vi "Configure Form Object.vi"(8 "error in (no error)":errorcluster, 10 "Table Name":string, 11 "Panel Form Controller in":refnum<class "Panel Form Controller.lvclass">) -> (0 "error out":errorcluster, 3 "Panel Form Controller out":refnum<class "Panel Form Controller.lvclass">)   [LabVIEW 2020]
uses:
  Database OOP/Table Libraries/Basic Table/Basic Table Class/Basic Table.lvclass
  Database OOP/Table Libraries/Table Configuration Interface/Table Configuration Interface.lvclass
  Panel Form Controller.lvclass
  C:/Program Files (x86)/National Instruments/LabVIEW 2020/vi.lib/MGI/Panel Manager/Panel Actor/Panel Actor/Panel Actor.lvclass
  C:/Program Files (x86)/National Instruments/LabVIEW 2020/vi.lib/MGI/Monitored Actor/Monitored Actor/Monitored Actor/Monitored Actor.lvclass
  C:/Program Files (x86)/National Instruments/LabVIEW 2020/vi.lib/ActorFramework/Actor/Actor.lvclass
  C:/Users/User/Desktop/Raman Program/Database OOP/source/Forms AF/Form Controller/Panel Form Controller.lvclass
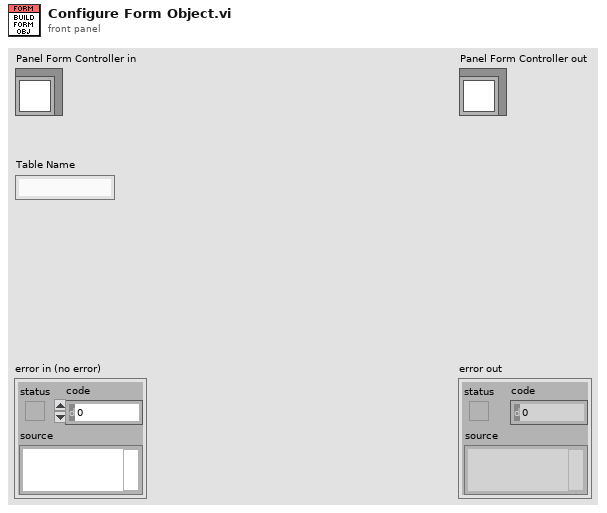
[diagram p1: front panel]
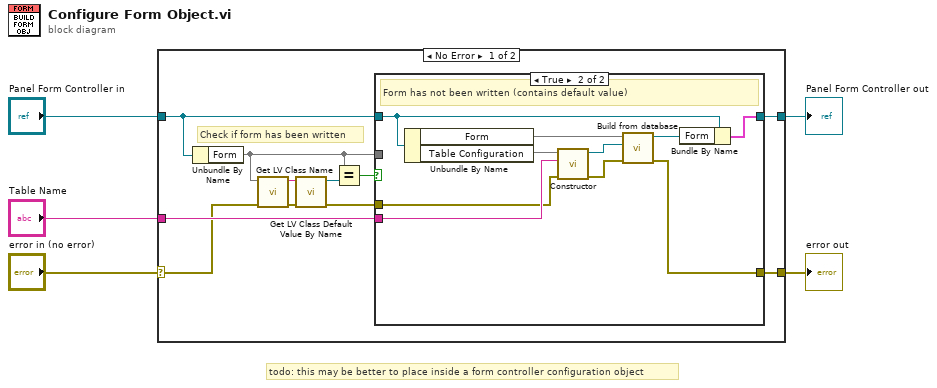
[diagram p0: block diagram]
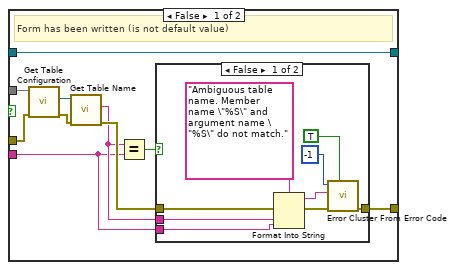
[diagram p2: hidden frame]
diagram:
  # "todo: this may be better to place inside a form controller configuration object"
  n1 = case shown="No Error" "error in (no error)" {
    selector: "error in (no error)" -> [w8 w48]
    tunnel: [w6 w48] -> w4
    tunnel: [w12 w47] -> w2
    tunnel: "Panel Form Controller in" -> [w13 w47]
    tunnel: "Table Name" -> [w10 _]
    frame No Error {
      # "Check if form has been written"
      n2 = Unbundle By Name(w13) -> ("Form"=w9)
      n3 = call <vilib>:"Get LV Class Name.vi"("error in (no error)"=w8, "object"=w9) -> ("error out"=w16:errorcluster, "class name"=w15:string)  [unwired: 8 in]
      n4 = call <vilib>:"Get LV Class Default Value By Name.vi"("error in (no error)"=w16, "class name"=w15) -> ("error out"=w7:errorcluster, "object"=w14:refnum<class>)  [unwired: 8 in]
      n5 = Equal?(x=w9, y=w14) -> (x = y?=w11:bool)
      n6 = case shown="True" w11 {
        tunnel: w13 -> [w24 w46]
        tunnel: [w24 w45] -> w12
        tunnel: w10 -> [w19 w43]
        tunnel: w9 -> [w26 _]
        tunnel: w7 -> [w25 w42]
        tunnel: [w18 w37] -> w6
        frame False {
          # "Form has been written (is not default value)"
          n7 = call "Get Table Configuration.vi"("error in (no error)"=w25, "Basic Table in"=w26) -> ("error out"=w17:errorcluster, "Table Configuration"=w23:refnum<class "Table Configuration Interface.lvclass">)  [unwired: 7 in, 1 out]
          n8 = call-dynamic "Get Table Name.vi"("error in (no error)"=w17, "Table Configuration Interface in"=w23) -> ("error out"=w21:errorcluster, "Table Name"=w20:string)  [unwired: 7 in, 1 out]
          n9 = Equal?(x=w20, y=w19) -> (x = y?=w22:bool)
          n10 = case shown="False" w22 {
            tunnel: w21 -> [w30 w36]
            tunnel: w20 -> [w29 _]
            tunnel: w19 -> [w28 _]
            tunnel: [w27 w36] -> w18
            frame False {
              n11 = Format Into String(format string="Ambiguous table name. Member name \"%S\" and argument name \"%S\" do not match.", error in=w30, w29, w28) -> (resulting string=w34:string, error out=w35:errorcluster)  [unwired: 1 in]
              n12 = call <vilib>:"Error Cluster From Error Code.vi"("show call chain? (False)"=TRUE, "error in (no error)"=w35, "error message (\"\")"=w34, "error code (0)"=-1) -> ("error out"=w27:errorcluster)  [unwired: 5 in]
            }
            frame True {
              # "Do nothing: form obj is valid and\nmatches form actor table name"
            }
          }
        }
        frame True {
          # "Form has not been written (contains default value)"
          n13 = Unbundle By Name(w46) -> ("Form"=w41, "Table Configuration"=w44)
          n14 = call-dynamic "Constructor.vi"("error in (no error)"=w42, "Table Name (Use Member Data)"=w43, "Table Configuration Interface in"=w44) -> ("error out"=w39:errorcluster, "Table Configuration Interface out"=w40:refnum<class "Table Configuration Interface.lvclass">)  [unwired: 7 in]
          n15 = call-dynamic "Build from database.vi"("error in (no error)"=w39, "Table Configuration"=w40, "Table in"=w41) -> ("error out"=w37:errorcluster, "Table out"=w38:refnum<class "Basic Table.lvclass">)  [unwired: 7 in]
          n16 = Bundle By Name(cluster=w46, "Form"=w38) -> (w45:cluster{})
        }
      }
    }
    frame Error {
    }
  }
  "error out" <- w4
  "Panel Form Controller out" <- w2
